vi "Unloading_scanned_Data_Event.vi"(0 "Unloading cyc Data":T1, 1 "Scanned  Data":string, 3 "error in":errorcluster) -> (7 "Scanned ?":bool, 10 "error out":errorcluster)   [LabVIEW 2017]
uses:
  Controls/Unloading_Cyc_Data.ctl
panel:
  out "second subarray":bool[](array[boolean])
  out "Boolean":bool
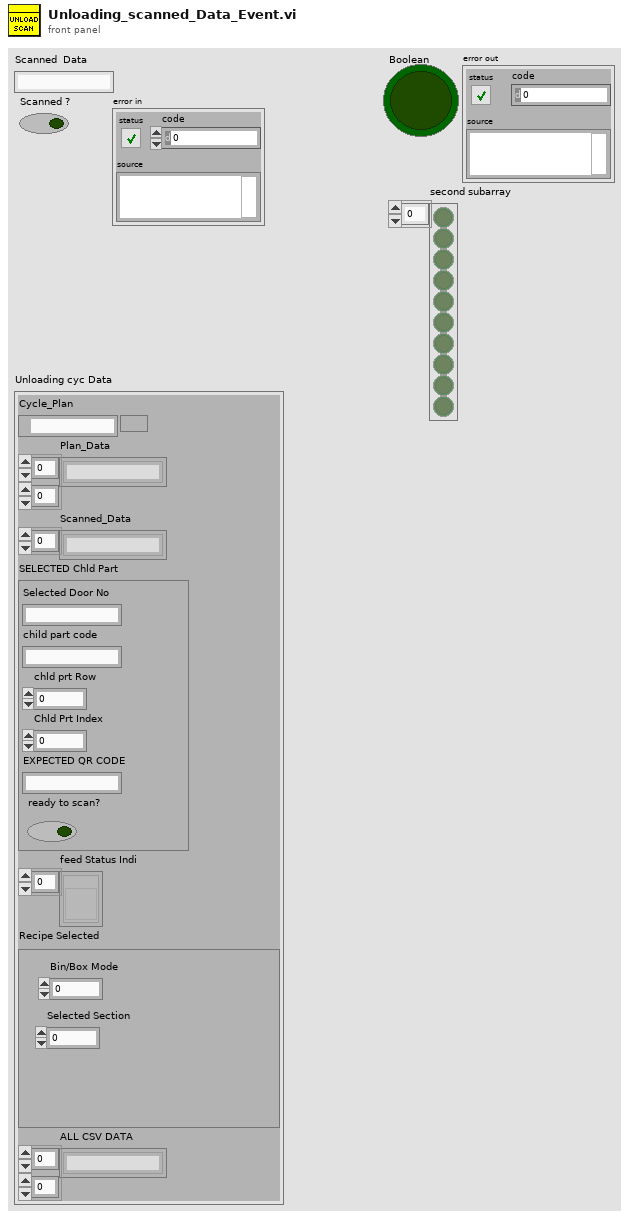
[diagram p1: front panel]
types:
  T1 = typedef "Unloading_Cyc_Data.ctl" = cluster{"Cycle_Plan":path, "Plan_Data":string[][], "Scanned_Data":string[], "SELECTED Chld Part":cluster{"Selected Door No":string, "child part code":string, "chld prt Row":i32, "Chld Prt Index":i32, "EXPECTED QR CODE":string, "ready to scan?":bool}, "feed Status Indi":refnum<vi>[], "Recipe Selected":cluster{"Bin/Box Mode":i32, "Selected Section":i32}, "ALL CSV DATA":string[][]}
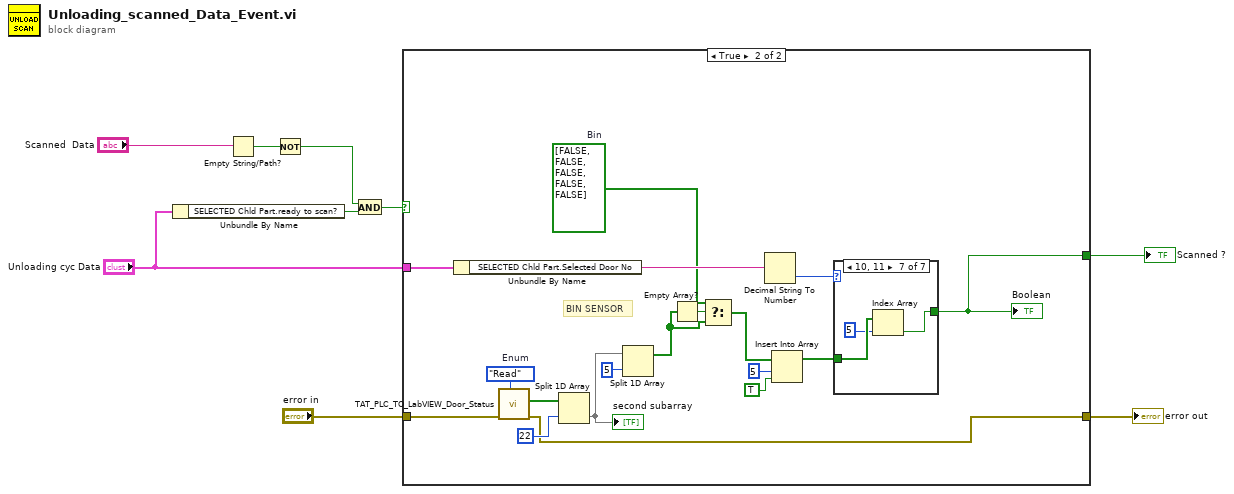
[diagram p0: block diagram]
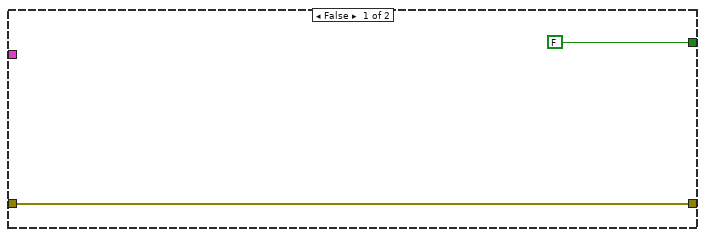
[diagram p2: hidden frame]
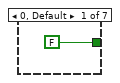
[diagram p3: hidden frame]
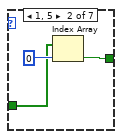
[diagram p4: hidden frame]
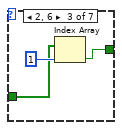
[diagram p5: hidden frame]
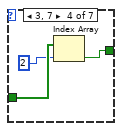
[diagram p6: hidden frame]
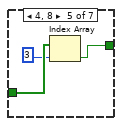
[diagram p7: hidden frame]
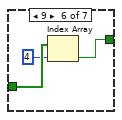
[diagram p8: hidden frame]
diagram:
  n1 = Unbundle By Name("Unloading cyc Data") -> ("SELECTED Chld Part.ready to scan?"=w8:bool)
  n2 = Empty String/Path?(string/path="Scanned  Data") -> (empty?=w4:bool)
  n3 = Not(x=w4) -> (.not. x?=w2:bool)
  n4 = And(x=w2, y=w8) -> (x .and. y?=w5:bool)
  n5 = case shown="True" w5 {
    tunnel: "Unloading cyc Data" -> [_ w28]
    tunnel: "error in" -> [w11 w21]
    tunnel: [w11 w20] -> w6
    tunnel: [FALSE w19] -> w1
    frame False {
    }
    frame True {
      w14 = bool[] [FALSE, FALSE, FALSE, FALSE, FALSE]  # Bin
      w26 = enum16{"Read", "Write"}."Read"  # Enum
      # "BIN SENSOR"
      n6 = Unbundle By Name(w28) -> ("SELECTED Chld Part.Selected Door No"=w27:string)
      n7 = call "TAT_PLC_TO_LabVIEW_Door_Status.vi"("Enum"=w26, "error in (no error)"=w21) -> ("error out"=w20:errorcluster, "Array 2"=w25:bool[])  [unwired: 8 in]
      n8 = Split 1D Array(array=w25, index=22) -> (second subarray=w23:bool[])  [unwired: 1 out]
      "second subarray" <- w23
      n9 = Split 1D Array(array=w23, index=5) -> (first subarray=w13:bool[])  [unwired: 1 out]
      n10 = Empty Array?(array=w13) -> (empty?=w18:bool)
      n11 = Select(t=w14, s=w18, f=w13) -> (s? t:f=w12:bool[])
      n12 = Decimal String To Number(string=w27) -> (number=w29:i32)  [unwired: 2 in, 1 out]
      n13 = Insert Into Array(array=w12, index=5, new element=TRUE) -> (w15:bool[])
      n14 = case shown="10, 11" w29 {
        tunnel: [FALSE w33 w34 w39 w42 w45 w48] -> w19
        tunnel: w15 -> [_ w31 w35 w38 w41 w44 w47]
        frame 0, Default {
        }
        frame 1, 5 {
          n15 = Index Array(array=w31, index=0) -> (element=w33:bool)
        }
        frame 2, 6 {
          n16 = Index Array(array=w35, index=1) -> (element=w34:bool)
        }
        frame 3, 7 {
          n17 = Index Array(array=w38, index=2) -> (element=w39:bool)
        }
        frame 4, 8 {
          n18 = Index Array(array=w41, index=3) -> (element=w42:bool)
        }
        frame 9 {
          n19 = Index Array(array=w44, index=4) -> (element=w45:bool)
        }
        frame 10, 11 {
          n20 = Index Array(array=w47, index=5) -> (element=w48:bool)
        }
      }
      "Boolean" <- w19
    }
  }
  "error out" <- w6
  "Scanned ?" <- w1
